vi "Store Static VI References for Subpanel.vi"(8 "error in (no error)":errorcluster, 11 "Server Config in":refnum<class "Server Config.lvclass">) -> (0 "error out":errorcluster, 3 "Server Config out":refnum<class "Server Config.lvclass">)   [LabVIEW 2016, in "Server Controller.lvlib" / "Server Config.lvclass"]
uses:
  Server Config.lvclass
  C:/Program Files (x86)/National Instruments/LabVIEW 2016/user.lib/Configuration Dialog Actor/Configuration.lvclass
  MAL-Framework/user.lib/Common Components/Msmt Configuration/Controller Configuration.lvclass
  <userlib>/Configuration Dialog Actor/Configuration.lvclass
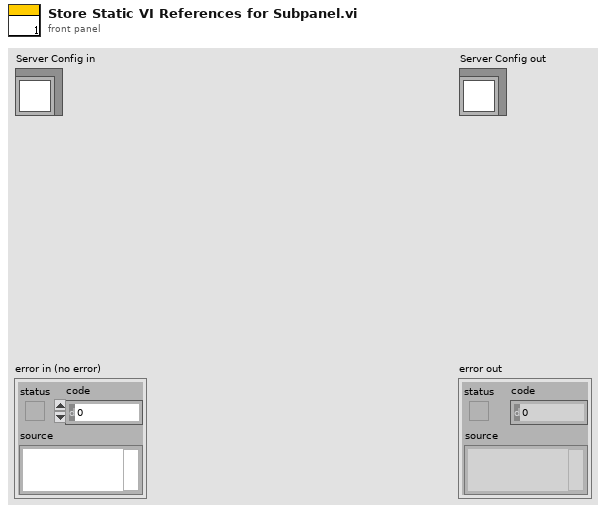
[diagram p1: front panel]
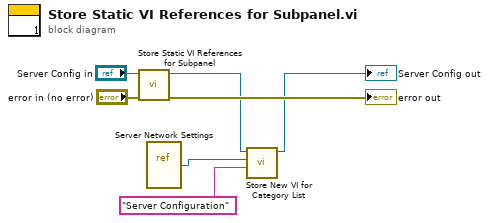
[diagram p0: block diagram]
diagram:
  n1 = call-parent "Store Static VI References for Subpanel.vi"("error in (no error)"="error in (no error)", "Controller Configuration in"="Server Config in") -> ("error out"=→"error out":errorcluster, "Controller Configuration out"=w4:refnum<class "Server Config.lvclass">)  [unwired: 8 in]
  n2 = vi-ref "Server Network Settings.vi"() -> (w2:refnum<vi>)
  n3 = call <userlib>:"Store New VI for Category List.vi"("String"="Server Configuration", "VI Refnum"=w2, "Configuration in"=w4) -> ("Configuration out"=→"Server Config out":refnum<class "Server Config.lvclass">)  [unwired: 7 in, 1 out]
